vi "Set Multi Gate Threshold Level [UML].vi"(6 "Gate Number":i32, 7 "Micropulse # In":i32, 8 "error in (no error)":errorcluster, 9 "Threshold":u16, 11 "Test Number":u32) -> (0 "error out":errorcluster, 5 "Micropulse # Out":i32)   [LabVIEW 2026, in "MicroPulse_Driver.lvlib"]
doc: "Multi-gate version of UPL command. Specifies the UPPER reporting threshold for the specified Test Number (Tn) and Gate Number (Gn). Any signals ABOVE the UML threshold level value and within the search gate area will be recognised by the signal processor as possible valid peaks, depending on HMS.\n\nParameters:\n<Tn> : Test number. An integer value from 0 to the maximum number of tests (default maximum is 1279 tests).\nTn = 0 for all conventional tests. If the S extension is used it applies to all tests in the sweep number specified: 1-32, 0 = all sweeps\n\n<Gn> : Gate Number, an integer value from 0 to 4.\nGn = 0 for all gates in the test\n\n<Value> : Integer between 10 and 255 ( 8-bit modes)\nInteger between 10 and 1023 (10-bit modes)\nInteger between 10 and 4095 (12-bit modes)\n\nNote:\nValid in Multi-gate Mode only (AMP 31 & 32)"
uses:
  MicroPulse_Driver.lvlib
  Private/MP-Registry Action-Enum.ctl
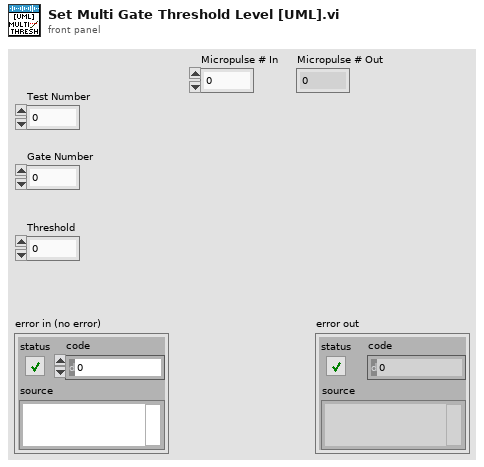
[diagram p1: front panel]
types:
  T1 = typedef "MicroPulse_Driver.lvlib/MP-Registry Action-Enum.ctl" = enum16{"Read", "Add Test", "Add Command", "Add Gate Command", "Add Encoder Command", "Clear Command  List", "Set Registry", "Set System Details", "Set DOF", "Set Velocity", "Disable Asynch Reads", "Enable Asynch Reads", "Add Connection", "Disconnect", "Shutdown"}
  T2 = typedef "Micropulse.lvlib/MP-Registry Data-Cluster.ctl" = cluster{"Instrument Type":T3, "Serial #":u64, "Sample Frequency":T4, "dt (us)":dbl, "DOF":T5, "Material Velocity":dbl, "Asynch Reads":T6, "NUM of Tests":u32, "System Details":T7, "Gates":T9[], "Encoders":T16[], "CMD LUT":variant, "Command List":string}
  T3 = typedef "Micropulse.lvlib/MP - instrument type.ctl" = enum16{"MicroPulse 5", "LT1", "LT2", "LTPA", "MPLT", "MicroPulse 6", "PipeScanner", "<MicroPulse>", "Micropulse 4", "Simulated Data"}
  T4 = typedef "Micropulse.lvlib/MP - sample frequency.ctl" = enum16{"Use Default", "200MHz (LT2 only)", "100MHz", "50MHz", "25MHz", "10MHz"}
  T5 = typedef "Micropulse.lvlib/MP - data output format.ctl" = enum16{"", "8-bit Mode", "10-bit Mode", "12-bit Mode", "16-bit Mode", "8-bit Log Mode", "12-bit Packed Mode"}
  T6 = typedef "Micropulse.lvlib/MP - asynch read mode.ctl" = enum16{"Disabled", "Enabled"}
  T7 = typedef "Micropulse.lvlib/MP - general system status.ctl" = cluster{"System Type":T3, "Serial No.":u64, "Channels":cluster{"Conv":u8, "PA":u16, "Extra":u32}, "Sample Frequency":cluster{"Default":u8, "Actual":u8}, "Software Versions":string, "Data Output Format":cluster{"Default":T5, "Actual":T5}, "Temperatures":cluster{"System":u8, "Processor":u8, "Slave Sys":u8, "Slave Proc":u8}, "Tx Buffer Size":u32, "System Error":string, "No. of Cards":u8, "DAC Gain":i16, "Uptimes":cluster{"since Power":u32, "since RSTS":u32, "since SRST":u32}, "Voltages":cluster{"Nominal":dbl, "Measured":dbl, "Difference":dbl}[], "Interface Cards":T8[]}
  T8 = typedef "Micropulse.lvlib/MP - interface card status.ctl" = cluster{"Status":u8, "Map":u8, "Board - T":u8, "FPGA - T":u8, "PAIF Status":string, "Version":string}
  T9 = typedef "Micropulse.lvlib/MP - Registry Gates.ctl" = cluster{"Display Gate":T10, "ETM Mode":T11, "Echo Gate":T12, "Insp Gates":T13[]}
  T10 = typedef "Micropulse.lvlib/MP - display gate.ctl" = cluster{"Start":dbl, "Length":dbl}
  T11 = typedef "Micropulse.lvlib/MP - echo gate mode.ctl" = enum16{"Echo Trigger OFF", "Echo Gate Display Mode", "Echo Trigger ON", "Multi Gate or FMC Mode", "Reserved", "PA - Echo Trigger ON"}
  T12 = typedef "Micropulse.lvlib/MP - echo gate parameters.ctl" = cluster{"Start (us)":dbl, "Length (us)":dbl, "Threshold":u16, "Colour":u32}
  T13 = typedef "Micropulse.lvlib/MP - multigate inspection gate parameters.ctl" = cluster{"Start (us)":dbl, "Length (us)":dbl, "Threshold":u16, "Enabled?":bool, "Max # Peaks":u16, "Hysteresis":T14, "Mode":T15, "Inverted?":bool, "Colour ":u32}
  T14 = typedef "Micropulse.lvlib/MP - hysteresis level.ctl" = enum16{"None", "3dB", "6dB", "9dB", "12dB"}
  T15 = typedef "Micropulse.lvlib/MP - multigate mode.ctl" = enum16{"1st Peak in Gate", "Largest Peak In Gate", "All Peaks In Gate", "1st Threshold Crossing"}
  T16 = typedef "Micropulse.lvlib/MP - encoder settings.ctl" = cluster{"Encoder Type":T17, "Counts/mm":u32, "Enable Termination?":bool, "Multiplier":u32, "Backlash Period (s)":dbl, "Encoder Filter":u32}
  T17 = typedef "Micropulse.lvlib/MP - encoder type.ctl" = enum16{"Quadrature", "Step/Direction"}
  T18 = typedef "Micropulse.lvlib/TCP config.ctl" = cluster{"Connection ID":refnum<k5>, "IP address":string, "host port":u16, "OC timeout":i32, "Read timeout":i32, "Write timeout":i32}
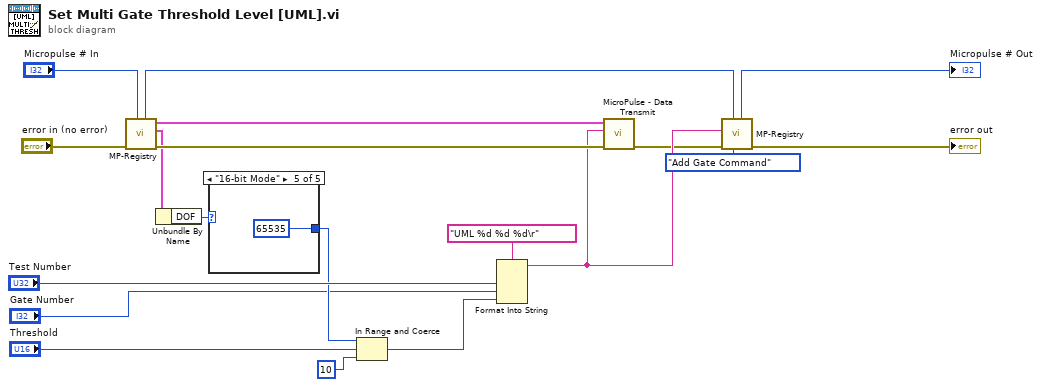
[diagram p0: block diagram]
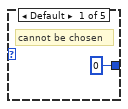
[diagram p2: hidden frame]
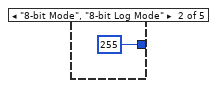
[diagram p3: hidden frame]
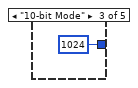
[diagram p4: hidden frame]
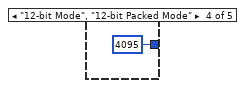
[diagram p5: hidden frame]
diagram:
  n1 = call "MP-Registry.vi"("Micropulse # In"="Micropulse # In", "error in (no error)"="error in (no error)") -> ("error out"=w17:errorcluster, "Micropulse Data"=w5:T2, "TCP config"=w16:T18, "Micropulse # Out"=w10:i32)  [unwired: 6 in]
  n2 = Unbundle By Name(w5) -> ("DOF"=w4:T5)
  n3 = case shown="\"16-bit Mode\"" w4 {
    tunnel: [u16 0 ("upper limit") u16 255 ("upper limit") u16 1024 ("upper limit") u16 4095 ("upper limit") u16 65535 ("upper limit")] -> w3
    frame Default {
      # "cannot be chosen"
    }
    frame "8-bit Mode", "8-bit Log Mode" {
    }
    frame "10-bit Mode" {
    }
    frame "12-bit Mode", "12-bit Packed Mode" {
    }
    frame "16-bit Mode" {
    }
  }
  n4 = In Range and Coerce(upper limit=w3, x="Threshold", lower limit=u16 10) -> (coerced(x)=w2:u16)  [unwired: 1 out]
  n5 = Format Into String(format string="UML %d %d %d\r", "Test Number", "Gate Number", w2) -> (resulting string=w14:string)  [unwired: 2 in, 1 out]
  n6 = call "MicroPulse - Data Transmit.vi"("error in (no error)"=w17, "data"=w14, "TCP config"=w16) -> ("error out"=w12:errorcluster)  [unwired: 6 in, 2 out]
  n7 = call "MP-Registry.vi"("Action"=MP-Registry_Action-Enum."Add Gate Command", "Micropulse # In"=w10, "error in (no error)"=w12, "Data in"=w14) -> ("error out"=→"error out":errorcluster, "Micropulse # Out"=→"Micropulse # Out":i32)  [unwired: 4 in, 2 out]
